vi "Update Map - Elimination.vi"(8 "Column":i32, 9 "Row":i32, 10 "Last Position":T1, 11 "map in":refnum<data-value>) -> (3 "map out":refnum<data-value>)   [LabVIEW 2015, in "DS Square.lvlib"]
uses:
  DS Square.lvlib
  Map.ctl
  Square Status.ctl
  Square State.ctl
  Center of Mass.ctl
  Common/Position.ctl
  SubVIs/Read-Only Globals.vi
  SubVIs/Globals (private).vi
  Square/Square.lvclass
  Common/Common.lvlib
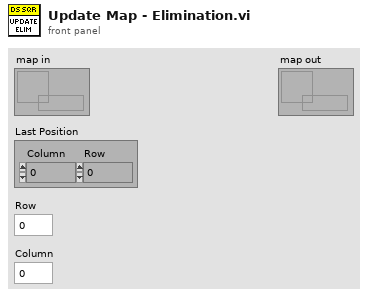
[diagram p1: front panel]
types:
  T1 = typedef "Common.lvlib/Position.ctl" = cluster{"Column":i32, "Row":i32}
  T2 = typedef "DS Square.lvlib/Square State.ctl" = enum16{"Unknown", "Empty", "Occupied - Active", "Occupied - Cool Down", "Attacked", "Enemy", "Enemy Wall"}
  T3 = typedef "DS Square.lvlib/Map.ctl" = cluster{"squares":T4[][], "center of mass":T5}
  T4 = typedef "DS Square.lvlib/Square Status.ctl" = cluster{"square state":T2, "probability":dbl, "last update":i32}
  T5 = typedef "DS Square.lvlib/Center of Mass.ctl" = cluster{"row":dbl, "col":dbl, "mass":dbl}
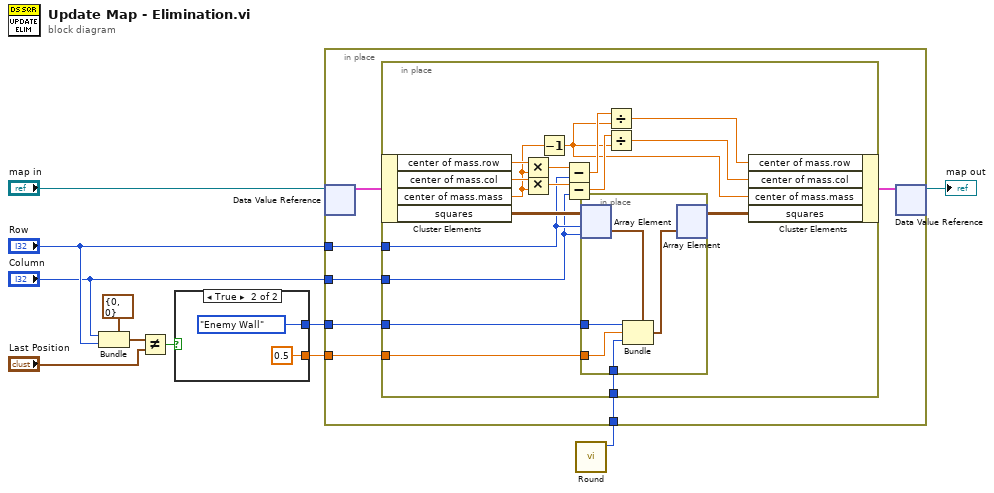
[diagram p0: block diagram]
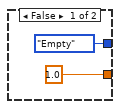
[diagram p2: hidden frame]
diagram:
  n1 = Bundle(cluster=T1 {"Column"=0, "Row"=0} ("Position in"), "Column"="Column", "Row"="Row") -> (w6:T1)
  n2 = Not Equal?(x=w6, y="Last Position") -> (x != y?=w5:bool)
  n3 = case shown="True" w5 {
    tunnel: [Square_State."Empty" ("square state") Square_State."Enemy Wall" ("square state")] -> w1
    tunnel: [1.0 ("probability") 0.5 ("probability")] -> w2
    frame False {
    }
    frame True {
    }
  }
  n4 = call "Round.vi"() -> ("Round"=w9:i32)  [unwired: 11 in]
  n5 = in-place {
    in-place-border: w9 -> [w22]
    in-place-border: "Row" -> [w21]
    in-place-border: "Column" -> [w20]
    in-place-border: w2 -> [w19]
    in-place-border: w1 -> [w18]
    n6 = in-place-dvr #1("map in") -> (w16:T3)  [unwired: 1 out]
    n7 = in-place {
      in-place-border: w22 -> [w39]
      in-place-border: w21 -> [w30]
      in-place-border: w20 -> [w29]
      in-place-border: w19 -> [w38]
      in-place-border: w18 -> [w37]
      n8 = in-place-cluster #2(w16) -> ("center of mass.row"=w33:dbl, "center of mass.col"=w34:dbl, "center of mass.mass"=w26:dbl, "squares"=w36:T4[][])
      n9 = Multiply(x=w33, y=w26) -> (x*y=w32:dbl)
      n10 = Multiply(x=w34, y=w26) -> (x*y=w31:dbl)
      n11 = Decrement(x=w26) -> (x-1=w23:dbl)
      n12 = Subtract(x=w32, y=w30) -> (x-y=w28:dbl)
      n13 = Subtract(x=w31, y=w29) -> (x-y=w27:dbl)
      n14 = in-place {
        in-place-border: w39 -> [w43]
        in-place-border: w38 -> [w41]
        in-place-border: w37 -> [w40]
        n15 = in-place-array #3(w36, w30, w29) -> (w44:T4)
        n16 = Bundle(cluster=w44, "square state"=w40, "probability"=w41, "last update"=w43) -> (w42:T4)
        n17 = in-place-array #3(w42) -> (w35:T4[][])  [unwired: 2 out]
      }
      n18 = Divide(x=w28, y=w23) -> (x/y=w25:dbl)
      n19 = Divide(x=w27, y=w23) -> (x/y=w24:dbl)
      n20 = in-place-cluster #2("center of mass.row"=w25, "center of mass.col"=w24, "center of mass.mass"=w23, "squares"=w35) -> (w17:T3)
    }
    n21 = in-place-dvr #1(w17) -> (→"map out":refnum<data-value>)  [unwired: 1 out]
  }
